vi "Correlation ID generator.vi"() -> (0 "Correlation ID":string)   [LabVIEW 2016]
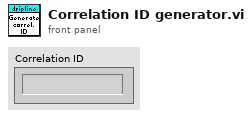
[diagram p1: front panel]
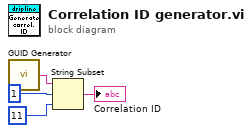
[diagram p0: block diagram]
diagram:
  n1 = call "GUID Generator.vi"() -> ("GUID"=w4:string)  [unwired: 9 in]
  n2 = String Subset(string=w4, offset (0)=1, length (rest)=11 ("length (rest)")) -> (substring=→"Correlation ID":string)
